vi "Write AppOutput.vi"(8 "error in (no error)":errorcluster, 10 "RingdownOutput":T1, 11 "VisualizeAppRingdown in":refnum<class "VisualizeAppRingdown.lvclass">) -> (0 "error out":errorcluster, 3 "VisualizeAppRingdown out":refnum<class "VisualizeAppRingdown.lvclass">)   [LabVIEW 2017, in "Visualization.lvlib" / "VisualizeAppRingdown.lvclass"]
uses:
  VisualizeAppRingdown.lvclass
  Modules/AppPlugins/RingdownPlugin/PublicAPI/TypeDef/RingdownOutput.ctl
  VisualizeAppRingdown.lvclass/VisualizeAppRingdown.ctl
  Modules/AppPlugins/RingdownPlugin/RingdownPlugin.lvclass
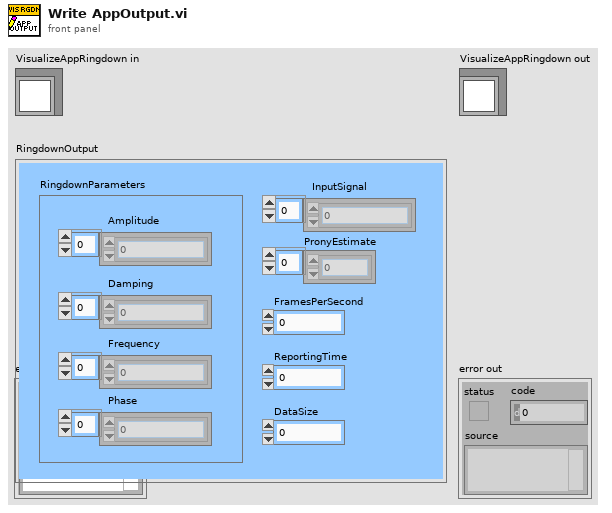
[diagram p1: front panel]
types:
  T1 = typedef "AppPlugins.lvlib/RingdownPlugin.lvclass/RingdownOutput.ctl" = cluster{"FramesPerSecond":dbl, "PronyEstimate":dbl[], "RingdownParameters":cluster{"Amplitude":dbl[], "Damping":dbl[], "Frequency":dbl[], "Phase":dbl[]}, "ReportingTime":dbl, "DataSize":u32, "InputSignal":dbl[]}
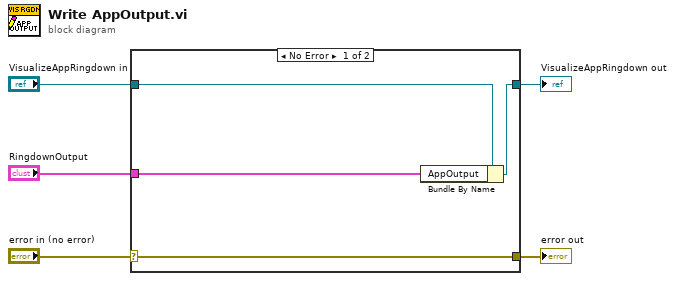
[diagram p0: block diagram]
diagram:
  n1 = case shown="No Error" "error in (no error)" {
    selector: "error in (no error)" -> [w9 w10]
    tunnel: [w9 w10] -> w4
    tunnel: [w7 w11] -> w2
    tunnel: "VisualizeAppRingdown in" -> [w8 w11]
    tunnel: "RingdownOutput" -> [w6 _]
    frame No Error {
      n2 = Bundle By Name(cluster=w8, "AppOutput"=w6) -> (w7:refnum<class "VisualizeAppRingdown.lvclass">)
    }
    frame Error {
    }
  }
  "error out" <- w4
  "VisualizeAppRingdown out" <- w2
